vi "build_boolean_array.vi"(2 "Off times":i32[](array[numeric]), 3 "On times":i32[](array[numeric])) -> (0 "max time":i32, 1 "Array":bool[][](array[boolean]))   [LabVIEW 2012]
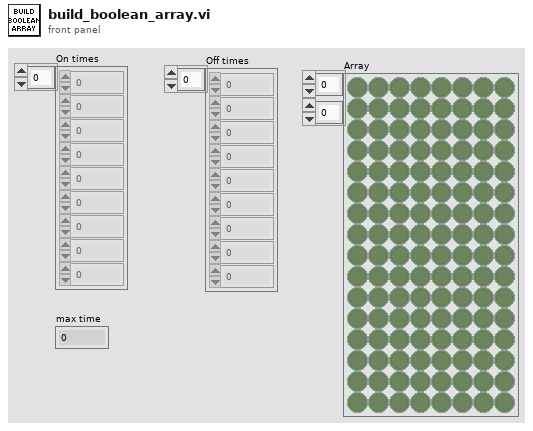
[diagram p1: front panel]
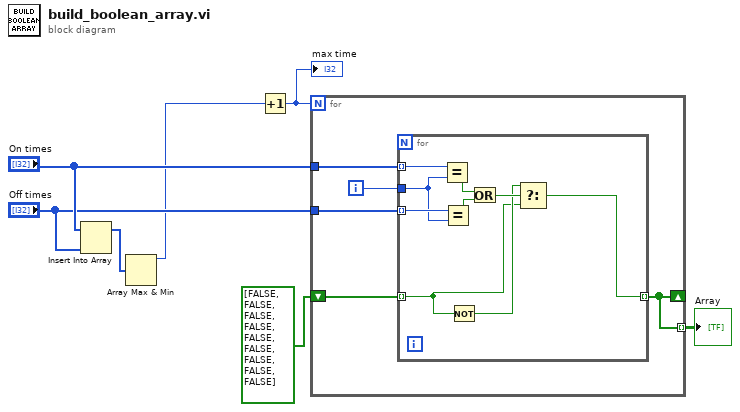
[diagram p0: block diagram]
diagram:
  n1 = Insert Into Array(array="On times", new element="Off times") -> (w7:i32[])  [unwired: 1 in]
  n2 = Array Max & Min(array=w7) -> (max value=w2:i32)  [unwired: 3 out]
  n3 = Increment(x=w2) -> (x+1=w1:i32)
  "max time" <- w1
  n4 = for {
    N: w1 -> [_]
    tunnel: "On times" -> [w12]
    tunnel: "Off times" -> [w11]
    shift-right: [w8] -> _
    shift-left: bool[] [FALSE, FALSE, FALSE, FALSE, FALSE, FALSE, FALSE, FALSE, FALSE] -> [w9]
    tunnel: [w8] -> w3 mode=indexing
    i -> [w10]
    n5 = for {
      tunnel: w12 -> [w21] mode=indexing
      tunnel: w11 -> [w20] mode=indexing
      tunnel: w10 -> [w17]
      tunnel: w9 -> [w14] mode=indexing
      tunnel: [w13] -> w8 mode=indexing
      n6 = Equal?(x=w21, y=w17) -> (x = y?=w18:bool)
      n7 = Equal?(x=w20, y=w17) -> (x = y?=w19:bool)
      n8 = Not(x=w14) -> (.not. x?=w15:bool)
      n9 = Or(x=w18, y=w19) -> (x .or. y?=w16:bool)
      n10 = Select(t=w15, s=w16, f=w14) -> (s? t:f=w13:bool)
    }
  }
  "Array" <- w3
